vi "ATSpectrograph_getEvent_reportedDisperserPosition.vi"(8 "error in (no error)":errorcluster, 11 "logevent_reportedDisperserPosition_Ctl":T1) -> (0 "error out":errorcluster, 2 "function return":i32, 3 "logevent_reportedDisperserPosition_Ctl out":T1)   [LabVIEW 2016, in "SALLV_ATSpectrograph.lvlib"]
doc: "int ATSpectrograph_shm_getEvent_reportedDisperserPositionLV(ATSpectrograph_logevent_reportedDisperserPositionLV *logevent_reportedDisperserPosition_Ctl );"
uses:
  SALLV_ATSpectrograph.lvlib
  DataTypes/logevent_reportedDisperserPosition.ctl
  SALLV_ATSpectrograph.so
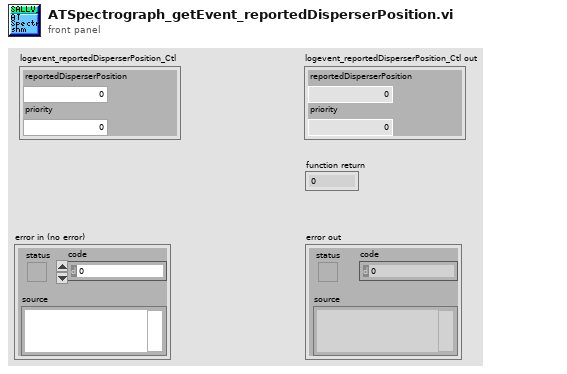
[diagram p1: front panel]
types:
  T1 = typedef "SALLV_ATSpectrograph.lvlib/logevent_reportedDisperserPosition.ctl" = cluster{"reportedDisperserPosition":i32, "priority":i32}
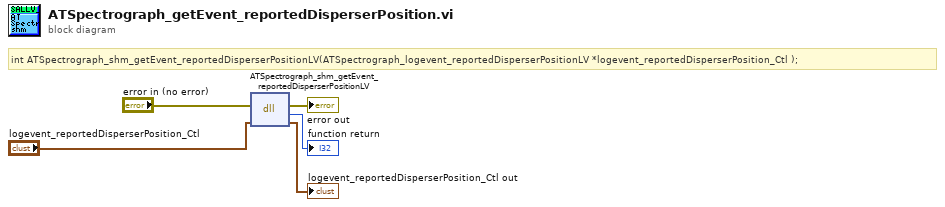
[diagram p0: block diagram]
diagram:
  # "int ATSpectrograph_shm_getEvent_reportedDisperserPositionLV(ATSpectrograph_logevent_reportedDisperserPositionLV *logevent_reportedDisperserPosition_Ctl );"
  n1 = dll-call lib="home/harini/TCS/develop/SALLV_ATSpectrograph/SALLV_ATSpectrograph.*" fn="ATSpectrograph_shm_getEvent_reportedDisperserPositionLV"(error in="error in (no error)", "logevent_reportedDisperserPosition_Ctl"="logevent_reportedDisperserPosition_Ctl") -> (error out=→"error out":errorcluster, →"function return":i32, "logevent_reportedDisperserPosition_Ctl"=→"logevent_reportedDisperserPosition_Ctl out":T1)  [unwired: 2 in, 1 out]
